vi "ReadFromConfigurationFile.vi"(8 "error in (no error)":errorcluster, 10 "Path":path, 11 "SMO.UI.MAUI in":refnum<class "SMO.UI.MAUI.lvclass">) -> (0 "error out":errorcluster, 2 "SpecificData":T1, 3 "SMO.UI.MAUI out":refnum<class "SMO.UI.MAUI.lvclass">)   [LabVIEW 2020, in "SMO.UI.MAUI.lvclass"]
uses:
  SMO.UI.MAUI.lvclass
  Typedefs/SpecificConfiguration.ctl
  <vilib>/Utility/config.llb/NI_LVConfig.lvlib
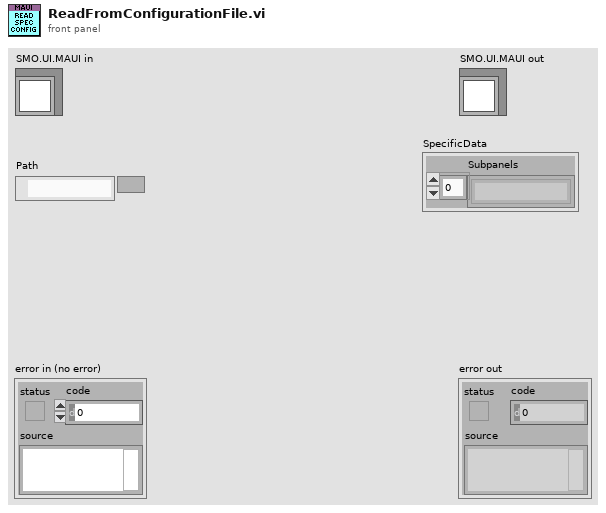
[diagram p1: front panel]
types:
  T1 = typedef "SMO.UI.MAUI.lvclass/SpecificConfiguration.ctl" = cluster{"Subpanels":string[]}
  T2 = typedef "NI_LVConfig.lvlib/Config Data RefNum.ctl" = refnum<k1>
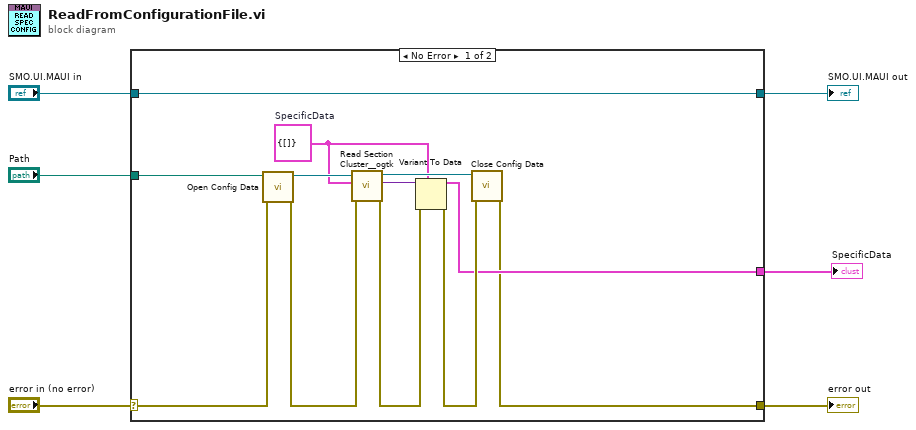
[diagram p0: block diagram]
diagram:
  n1 = case shown="No Error" "error in (no error)" {
    selector: "error in (no error)" -> [w14 w20]
    tunnel: [w7 w20] -> w5
    tunnel: [w18 w19] -> w3
    tunnel: "SMO.UI.MAUI in" -> [w18 w19]
    tunnel: "Path" -> [w16 _]
    tunnel: [w8 _] -> w1
    frame No Error {
      w11 = T1 {"Subpanels"=[]}  # SpecificData
      n2 = call <vilib>:"Open Config Data.vi"("error in (no error)"=w14, "configuration file path"=w16) -> ("error out"=w13:errorcluster, "refnum"=w17:T2)  [unwired: 7 in, 1 out]
      n3 = call <userlib>:"Read Section Cluster__ogtk.vi"("error in (no error)"=w13, "Section Formatted Cluster Type"=w11, "refnum"=w17) -> ("error out"=w10:errorcluster, "Section Formatted Cluster"=w12:variant, "dup refnum"=w15:T2)  [unwired: 4 in, 2 out]
      n4 = Variant To Data(error in=w10, type=w11, Variant=w12) -> (data=w8:T1, error out=w9:errorcluster)
      n5 = call <vilib>:"Close Config Data.vi"("error in (no error)"=w9, "refnum"=w15) -> ("error out"=w7:errorcluster)  [unwired: 8 in, 1 out]
    }
    frame Error {
    }
  }
  "error out" <- w5
  "SMO.UI.MAUI out" <- w3
  "SpecificData" <- w1
